vi "PicoScope2000aGetRapidBlock.vi"(0 "error in":errorcluster, 5 "enabled array":i16[](array[numeric]), 7 "handle in":i16, 9 "Buffer and Transfer Settings":T1={"startIndex"=0, "Samples"=1000, "Down Sample Ratio"=2, "Down-Sample Mode"=0} {"Down-Sample Mode" items=["None"=0, "Aggregate"=1, "Decimate"=2, "Average"=4]; "Samples" format="%_6p"}, 11 "Rapid Block Acquisition Settings":T3={"preTriggerSamples"=0, "postTriggerSamples"=1000, "timebase"=2, "Oversample"=1, "Number of Captures"=1}, 12 "Device Info":T2) -> (1 "Channel A Buffer":i16[][](array[numeric]), 2 "Channel B Buffer":i16[][](array[numeric]), 3 "Channel D Buffer":i16[][](array[numeric]), 4 "error out":errorcluster, 6 "handle out":i16, 8 "Port 1":i16[][](array[numeric]), 10 "noOfSamples":u32[](array[numeric]), 13 "Channel C Buffer":i16[][](array[numeric]), 14 "Port 0":i16[][](array[numeric]), 15 "Overflow (binary)":i16[](array[numeric]) format="%06b")   [LabVIEW 2016]
doc: "This VI gets a set of blocks captured using rapid block mode. It outputs two-dimensional arrays for each channel that contain data from all the requested captures."
uses:
  ps2000a.dll
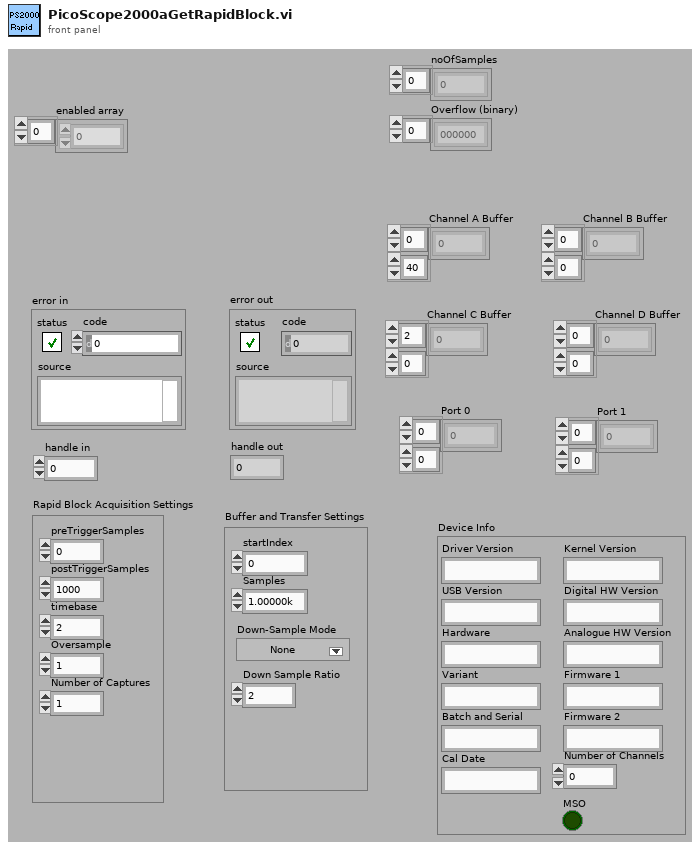
[diagram p1: front panel]
types:
  T1 = cluster{"startIndex":u64, "Samples":u64, "Down Sample Ratio":u64, "Down-Sample Mode":u32}
  T2 = cluster{"Driver Version":string, "USB Version":string, "Hardware":string, "Variant":string, "Batch and Serial":string, "Cal Date":string, "Kernel Version":string, "Digital HW Version":string, "Analogue HW Version":string, "Firmware 1":string, "Firmware 2":string, "MSO":bool, "Number of Channels":i16}
  T3 = cluster{"preTriggerSamples":u32, "postTriggerSamples":u32, "timebase":u32, "Oversample":i16, "Number of Captures":u32}
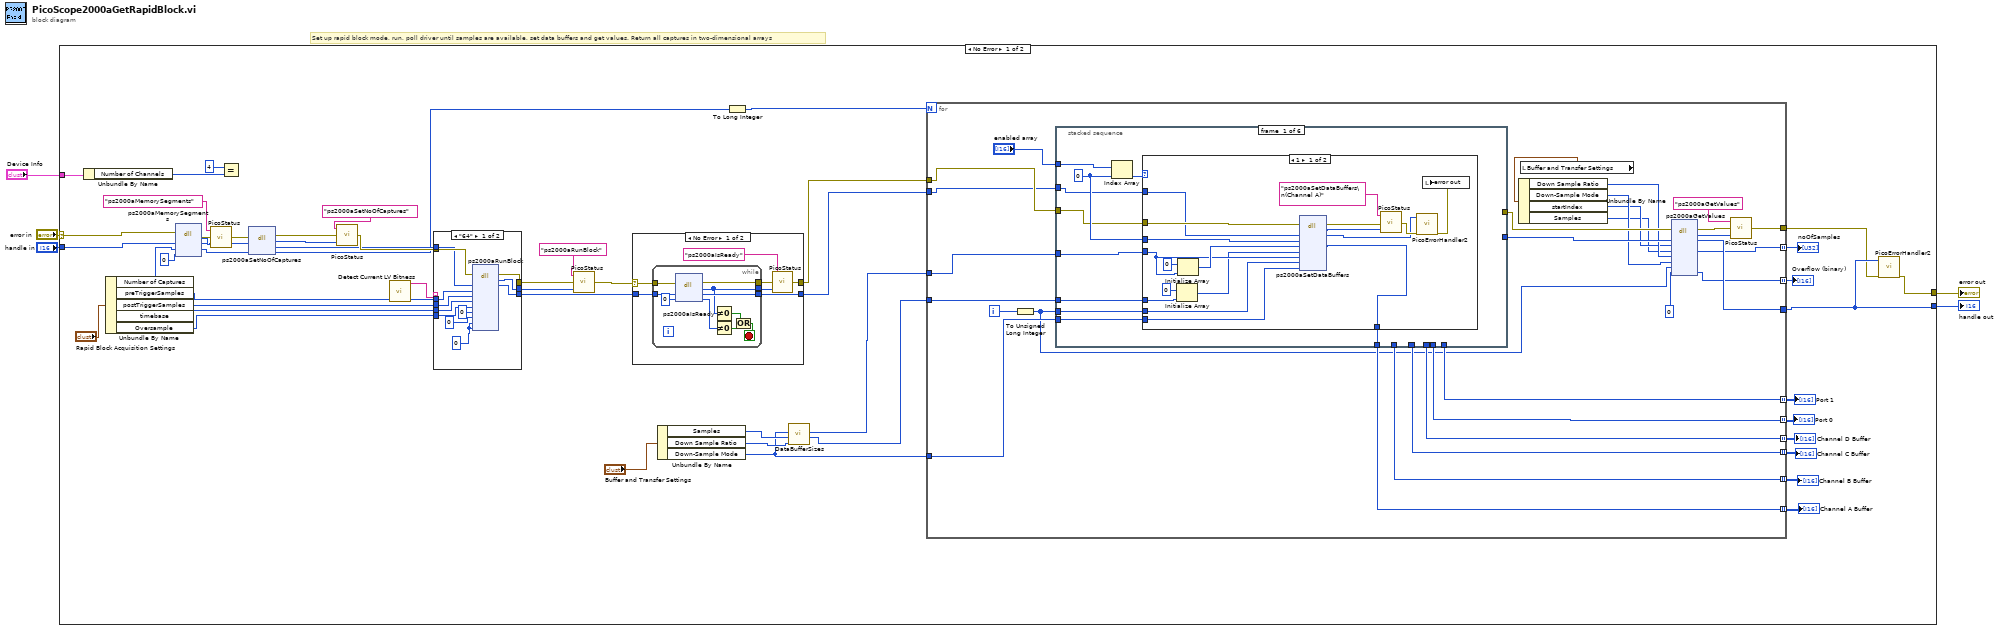
[diagram p0: block diagram]
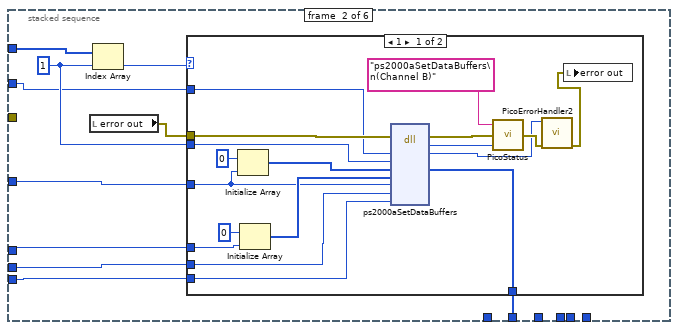
[diagram p3: hidden frame]
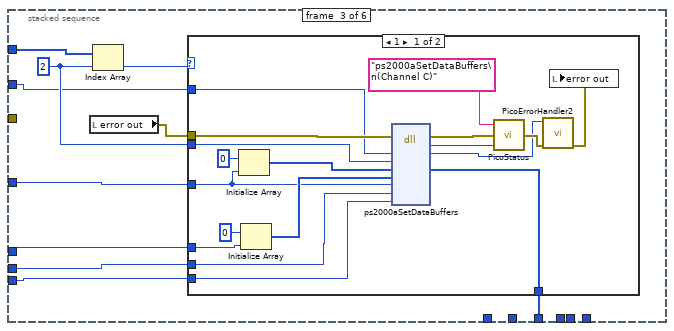
[diagram p5: hidden frame]
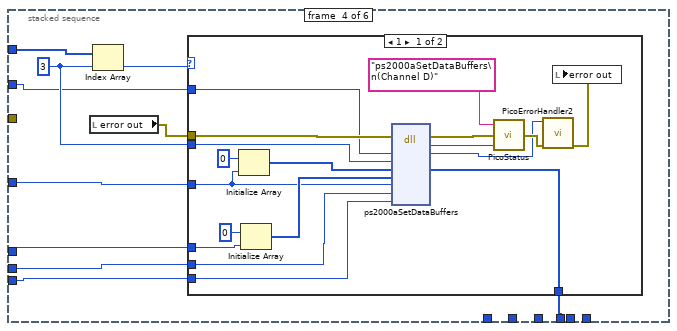
[diagram p7: hidden frame]
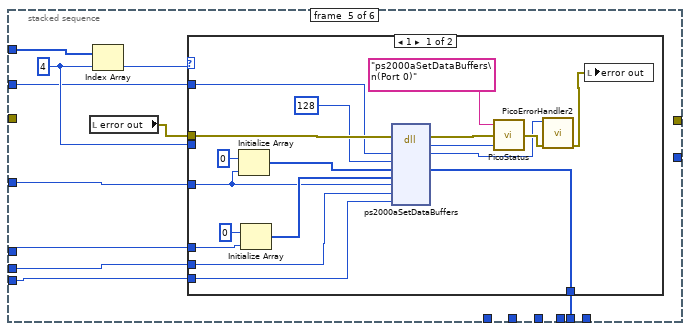
[diagram p9: hidden frame]
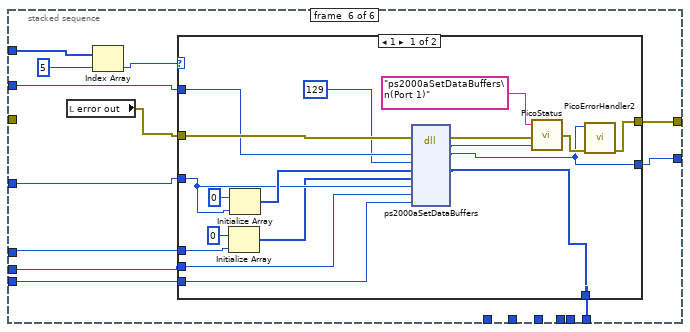
[diagram p11: hidden frame]
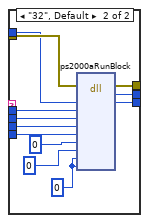
[diagram p13: hidden frame]
diagram:
  # "Set up rapid block mode, run, poll driver until samples are available, set data buffers and get values. Return all captures in two-dimensional arrays"
  n1 = case shown="No Error" "error in" {
    selector: "error in" -> [w45 w301]
    tunnel: [w26 w301] -> w4
    tunnel: "handle in" -> [w44 w300]
    tunnel: [w15 w300] -> w2
    tunnel: "Device Info" -> [w30 _]
    frame No Error {
      n2 = Unbundle By Name(w30) -> ("Number of Channels"=w29:i16)
      n3 = Unbundle By Name("Rapid Block Acquisition Settings") -> ("Number of Captures"=w40:u32, "preTriggerSamples"=w52:u32, "postTriggerSamples"=w51:u32, "timebase"=w53:u32, "Oversample"=w46:i16)
      n4 = dll-call lib="ps2000a.dll" fn="ps2000aMemorySegments" ("ps3000.dll:_ps3000_open_unit@0")(error in=w45, "handle"=w44, "nSegments"=w40, "nMaxSamples"=u32 0) -> (error out=w42:errorcluster, "PICO_STATUS"=w43:i32, "handle"=w37:i16, "nSegments"=w38:u32)  [unwired: 3 in, 1 out]
      n5 = call "PicoStatus.vi"("PICO STATUS"=w43, "error in"=w42, "source"="ps2000aMemorySegments") -> ("error out"=w36:errorcluster)
      n6 = Equal?(x=i16 4, y=w29) -> ()  [unwired: 1 out]
      n7 = dll-call lib="ps2000a.dll" fn="ps2000aSetNoOfCaptures" ("ps3000.dll:_ps3000_open_unit@0")(error in=w36, "handle"=w37, "nCaptures"=w38) -> (error out=w34:errorcluster, "PICO_STATUS"=w35:i32, "handle"=w31:i16, "nCaptures"=w16:u16)  [unwired: 2 in, 1 out]
      n8 = call "PicoStatus.vi"("PICO STATUS"=w35, "error in"=w34, "source"="ps2000aSetNoOfCaptures") -> ("error out"=w32:errorcluster)
      n9 = call "Detect Current LV Bitness.vi"() -> ("bitness"=w27:string)  [unwired: 11 in]
      n10 = case shown="\"64\"" w27 {
        tunnel: [w260 w280] -> w55
        tunnel: w53 -> [w263 w279]
        tunnel: w52 -> [w266 w278]
        tunnel: w51 -> [w265 w277]
        tunnel: [w261 w276] -> w50
        tunnel: [w262 w275] -> w49
        tunnel: w46 -> [w264 w274]
        tunnel: w32 -> [w268 w273]
        tunnel: w31 -> [w267 w272]
        frame "64" {
          w257 = u64 0 ("pParameter")
          n11 = dll-call lib="ps2000a.dll" fn="ps2000aRunBlock" ("ps3000.dll:_ps3000_open_unit@0")(error in=w268, "handle"=w267, "preTriggerSamples"=w266, "postTriggerSamples"=w265, "timebase"=w263, "oversample"=w264, "timeindisposed"=0, "segmentIndex"=u32 0, "lpReady"=w257, "pParameter"=w257) -> (error out=w262:errorcluster, "PICO_STATUS"=w261:i32, "handle"=w260:i16)  [unwired: 10 in, 1 out]
        }
        frame "32", Default {
          w269 = u32 0 ("pParameter")
          n12 = dll-call lib="ps2000a.dll" fn="ps2000aRunBlock" ("ps3000.dll:_ps3000_open_unit@0")(error in=w273, "handle"=w272, "preTriggerSamples"=w278, "postTriggerSamples"=w277, "timebase"=w279, "oversample"=w274, "timeindisposed"=0, "segmentIndex"=u32 0, "lpReady"=w269, "pParameter"=w269) -> (error out=w275:errorcluster, "PICO_STATUS"=w276:i32, "handle"=w280:i16)  [unwired: 10 in, 1 out]
        }
      }
      n13 = call "PicoStatus.vi"("PICO STATUS"=w50, "error in"=w49, "source"="ps2000aRunBlock") -> ("error out"=w48:errorcluster)
      n14 = case shown="No Error" w48 {
        selector: w48 -> [w285 w298]
        tunnel: w55 -> [w287 w299]
        tunnel: [w286 w299] -> w22
        tunnel: [w284 w298] -> w23
        frame No Error {
          n15 = while {
            tunnel: [w297] -> w286
            tunnel: w287 -> [w296]
            tunnel: [w291] -> w282
            tunnel: w285 -> [w290]
            tunnel: [w289] -> w283
            stop <- w295 stop-if-true
            n16 = dll-call lib="ps2000a.dll" fn="ps2000aIsReady" ("ps3000.dll:_ps3000_open_unit@0")(error in=w290, "handle"=w296, "ready"=i16 0) -> (error out=w289:errorcluster, "status"=w291:i32, "handle"=w297:i16, "ready"=w292:i16)  [unwired: 2 in, 1 out]
            n17 = Not Equal To 0?(x=w291) -> (x != 0?=w293:bool)
            n18 = Not Equal To 0?(x=w292) -> (x != 0?=w294:bool)
            n19 = Or(x=w293, y=w294) -> (x .or. y?=w295:bool)
          }
          n20 = call "PicoStatus.vi"("PICO STATUS"=w282, "error in"=w283, "source"="ps2000aIsReady") -> ("error out"=w284:errorcluster)
        }
        frame Error {
        }
      }
      n21 = Unbundle By Name("Buffer and Transfer Settings") -> ("Samples"=w24:u64, "Down Sample Ratio"=w19:u64, "Down-Sample Mode"=w18:u32)
      n22 = To Long Integer(number=w16) -> (32bit integer=w17:i32)
      n23 = call "DataBufferSizes.vi"("Down Sample Ratio"=w19, "Number of Samples"=w24, "Down-Sample Mode"=w18) -> ("min Buffer Size"=w21:i32, "Max Buffer Size"=w20:i32)  [unwired: 7 in]
      n24 = for {
        N: w17 -> [_]
        tunnel: w22 -> [w81]
        tunnel: w23 -> [w82]
        tunnel: w20 -> [w83]
        tunnel: w21 -> [w80]
        tunnel: w18 -> [w79]
        tunnel: [w75] -> w15
        tunnel: [w74] -> w7 mode=indexing
        tunnel: [w73] -> w14 mode=indexing
        tunnel: [w72] -> w13 mode=indexing
        tunnel: [w71] -> w12 mode=indexing
        tunnel: [w70] -> w11 mode=indexing
        tunnel: [w69] -> w10 mode=indexing
        tunnel: [w68] -> w9 mode=indexing
        tunnel: [w64] -> w8
        tunnel: [w58] -> w6 mode=indexing
        i -> [w65]
        n25 = To Unsigned Long Integer(number=w65) -> (unsigned 32bit integer=w62:u32)
        n26 = stacked-sequence {
          tunnel: "enabled array" -> [w93 w121 w149 w177 w205 w235]
          tunnel: w82 -> [w91 _ _ _ _ _]
          tunnel: w81 -> [w90 w119 w147 w175 w197 w232]
          tunnel: w83 -> [w87 w118 w146 w174 w204 w229]
          tunnel: [w89 _ _ _ _ _] -> w73
          tunnel: w62 -> [w88 w117 w145 w173 w203 w231]
          tunnel: [_ w116 _ _ _ _] -> w72
          tunnel: [_ _ w141 _ _ _] -> w71
          tunnel: [_ _ _ w169 _ _] -> w70
          tunnel: [_ _ _ _ w199 _] -> w69
          tunnel: [_ _ _ _ _ w228] -> w68
          tunnel: w80 -> [w86 w114 w143 w171 w201 w230]
          tunnel: w79 -> [w85 w113 w142 w170 w200 w227]
          tunnel: [_ _ _ _ _ w226] -> w67
          tunnel: [_ _ _ _ _ w225] -> w66
          frame #0 {
            w94 = 0 ("dimension size")
            n27 = Index Array(array=w93, index=w94) -> (element=w92:i16)
            n28 = case shown="1" w92 {
              tunnel: w94 -> [w106 _]
              tunnel: w91 -> [w108 _]
              tunnel: w90 -> [w107 _]
              tunnel: w87 -> [w104 _]
              tunnel: [w99 _] -> w89
              tunnel: w88 -> [w103 _]
              tunnel: w86 -> [w98 _]
              tunnel: w85 -> [w95 _]
              frame 1 {
                n29 = Initialize Array(i16 0 ("element"), w98) -> (w97:i16[])
                n30 = Initialize Array(i16 0 ("element"), w104) -> (w105:i16[])
                n31 = dll-call lib="ps2000a.dll" fn="ps2000aSetDataBuffers" ("ps3000.dll:_ps3000_open_unit@0")(error in=w108, "handle"=w107, "channel"=w106, "bufferMax"=w105, "bufferMin"=w97, "bufferLth"=w104, "segmentIndex"=w103, "downSampleRatioMode"=w95) -> (error out=w102:errorcluster, "PICO_STATUS"=w101:i32, "handle"=w100:i16, "bufferMax"=w99:i16[])  [unwired: 7 in, 1 out]
                n32 = call "PicoStatus.vi"("PICO STATUS"=w101, "error in"=w102, "source"="ps2000aSetDataBuffers\n(Channel A)") -> ("error out"=w111:errorcluster)
                n33 = call "PicoErrorHandler2.vi"("error in (no error)"=w111, "handle In"=w100) -> ("error out"=w110:errorcluster)  [unwired: 9 in]
                n34 = local write "error out"(w110) -> ()
              }
              frame 0, Default {
              }
            }
          }
          frame #1 {
            w122 = 1 ("dimension size")
            n35 = local read "error out"() -> (w115:errorcluster)
            n36 = Index Array(array=w121, index=w122) -> (element=w120:i16)
            n37 = case shown="1" w120 {
              tunnel: w122 -> [w126 _]
              tunnel: w115 -> [w131 _]
              tunnel: w119 -> [w123 _]
              tunnel: w118 -> [w129 _]
              tunnel: [w125 _] -> w116
              tunnel: w117 -> [w130 _]
              tunnel: w114 -> [w128 _]
              tunnel: w113 -> [w124 _]
              frame 1 {
                n38 = Initialize Array(i16 0 ("element"), w129) -> (w138:i16[])
                n39 = Initialize Array(i16 0 ("element"), w128) -> (w137:i16[])
                n40 = dll-call lib="ps2000a.dll" fn="ps2000aSetDataBuffers" ("ps3000.dll:_ps3000_open_unit@0")(error in=w131, "handle"=w123, "channel"=w126, "bufferMax"=w138, "bufferMin"=w137, "bufferLth"=w129, "segmentIndex"=w130, "downSampleRatioMode"=w124) -> (error out=w135:errorcluster, "PICO_STATUS"=w133:i32, "handle"=w132:i16, "bufferMax"=w125:i16[])  [unwired: 7 in, 1 out]
                n41 = call "PicoStatus.vi"("PICO STATUS"=w133, "error in"=w135, "source"="ps2000aSetDataBuffers\n(Channel B)") -> ("error out"=w139:errorcluster)
                n42 = call "PicoErrorHandler2.vi"("error in (no error)"=w139, "handle In"=w132) -> ("error out"=w140:errorcluster)  [unwired: 9 in]
                n43 = local write "error out"(w140) -> ()
              }
              frame 0, Default {
              }
            }
          }
          frame #2 {
            w150 = 2 ("dimension size")
            n44 = local read "error out"() -> (w144:errorcluster)
            n45 = Index Array(array=w149, index=w150) -> (element=w148:i16)
            n46 = case shown="1" w148 {
              tunnel: w150 -> [w154 _]
              tunnel: w144 -> [w159 _]
              tunnel: w147 -> [w151 _]
              tunnel: w146 -> [w157 _]
              tunnel: [w153 _] -> w141
              tunnel: w145 -> [w158 _]
              tunnel: w143 -> [w156 _]
              tunnel: w142 -> [w152 _]
              frame 1 {
                n47 = Initialize Array(i16 0 ("element"), w157) -> (w166:i16[])
                n48 = Initialize Array(i16 0 ("element"), w156) -> (w165:i16[])
                n49 = dll-call lib="ps2000a.dll" fn="ps2000aSetDataBuffers" ("ps3000.dll:_ps3000_open_unit@0")(error in=w159, "handle"=w151, "channel"=w154, "bufferMax"=w166, "bufferMin"=w165, "bufferLth"=w157, "segmentIndex"=w158, "downSampleRatioMode"=w152) -> (error out=w163:errorcluster, "PICO_STATUS"=w161:i32, "handle"=w160:i16, "bufferMax"=w153:i16[])  [unwired: 7 in, 1 out]
                n50 = call "PicoStatus.vi"("PICO STATUS"=w161, "error in"=w163, "source"="ps2000aSetDataBuffers\n(Channel C)") -> ("error out"=w167:errorcluster)
                n51 = call "PicoErrorHandler2.vi"("error in (no error)"=w167, "handle In"=w160) -> ("error out"=w168:errorcluster)  [unwired: 9 in]
                n52 = local write "error out"(w168) -> ()
              }
              frame 0, Default {
              }
            }
          }
          frame #3 {
            w178 = 3 ("dimension size")
            n53 = local read "error out"() -> (w172:errorcluster)
            n54 = Index Array(array=w177, index=w178) -> (element=w176:i16)
            n55 = case shown="1" w176 {
              tunnel: w178 -> [w182 _]
              tunnel: w172 -> [w187 _]
              tunnel: w175 -> [w179 _]
              tunnel: w174 -> [w185 _]
              tunnel: [w181 _] -> w169
              tunnel: w173 -> [w186 _]
              tunnel: w171 -> [w184 _]
              tunnel: w170 -> [w180 _]
              frame 1 {
                n56 = Initialize Array(i16 0 ("element"), w185) -> (w194:i16[])
                n57 = Initialize Array(i16 0 ("element"), w184) -> (w193:i16[])
                n58 = dll-call lib="ps2000a.dll" fn="ps2000aSetDataBuffers" ("ps3000.dll:_ps3000_open_unit@0")(error in=w187, "handle"=w179, "channel"=w182, "bufferMax"=w194, "bufferMin"=w193, "bufferLth"=w185, "segmentIndex"=w186, "downSampleRatioMode"=w180) -> (error out=w191:errorcluster, "PICO_STATUS"=w189:i32, "handle"=w188:i16, "bufferMax"=w181:i16[])  [unwired: 7 in, 1 out]
                n59 = call "PicoStatus.vi"("PICO STATUS"=w189, "error in"=w191, "source"="ps2000aSetDataBuffers\n(Channel D)") -> ("error out"=w195:errorcluster)
                n60 = call "PicoErrorHandler2.vi"("error in (no error)"=w195, "handle In"=w188) -> ("error out"=w196:errorcluster)  [unwired: 9 in]
                n61 = local write "error out"(w196) -> ()
              }
              frame 0, Default {
              }
            }
          }
          frame #4 {
            w206 = 4 ("dimension size")
            n62 = local read "error out"() -> (w202:errorcluster)
            n63 = Index Array(array=w205, index=w206) -> (element=w198:i16)
            n64 = case shown="1" w198 {
              tunnel: w206 -> [_ _]
              tunnel: w202 -> [w215 _]
              tunnel: w204 -> [w213 _]
              tunnel: [w210 _] -> w199
              tunnel: w203 -> [w214 _]
              tunnel: w201 -> [w212 _]
              tunnel: w200 -> [w209 _]
              tunnel: w197 -> [w207 _]
              frame 1 {
                n65 = Initialize Array(i16 0 ("element"), w213) -> (w222:i16[])
                n66 = Initialize Array(i16 0 ("element"), w212) -> (w221:i16[])
                n67 = dll-call lib="ps2000a.dll" fn="ps2000aSetDataBuffers" ("ps3000.dll:_ps3000_open_unit@0")(error in=w215, "handle"=w207, "channel"=128, "bufferMax"=w222, "bufferMin"=w221, "bufferLth"=w213, "segmentIndex"=w214, "downSampleRatioMode"=w209) -> (error out=w219:errorcluster, "PICO_STATUS"=w217:i32, "handle"=w216:i16, "bufferMax"=w210:i16[])  [unwired: 7 in, 1 out]
                n68 = call "PicoStatus.vi"("PICO STATUS"=w217, "error in"=w219, "source"="ps2000aSetDataBuffers\n(Port 0)") -> ("error out"=w223:errorcluster)
                n69 = call "PicoErrorHandler2.vi"("error in (no error)"=w223, "handle In"=w216) -> ("error out"=w224:errorcluster)  [unwired: 9 in]
                n70 = local write "error out"(w224) -> ()
              }
              frame 0, Default {
              }
            }
          }
          frame #5 {
            n71 = local read "error out"() -> (w234:errorcluster)
            n72 = Index Array(array=w235, index=5 ("dimension size")) -> (element=w233:i16)
            n73 = case shown="1" w233 {
              tunnel: w234 -> [w251 w256]
              tunnel: w232 -> [w250 w255]
              tunnel: w229 -> [w248 _]
              tunnel: [w244 _] -> w228
              tunnel: w231 -> [w247 _]
              tunnel: w230 -> [w243 _]
              tunnel: [w240 w256] -> w226
              tunnel: [w239 w255] -> w225
              tunnel: w227 -> [w237 _]
              frame 1 {
                n74 = Initialize Array(i16 0 ("element"), w243) -> (w242:i16[])
                n75 = Initialize Array(i16 0 ("element"), w248) -> (w249:i16[])
                n76 = dll-call lib="ps2000a.dll" fn="ps2000aSetDataBuffers" ("ps3000.dll:_ps3000_open_unit@0")(error in=w251, "handle"=w250, "channel"=129, "bufferMax"=w249, "bufferMin"=w242, "bufferLth"=w248, "segmentIndex"=w247, "downSampleRatioMode"=w237) -> (error out=w246:errorcluster, "PICO_STATUS"=w245:u32, "handle"=w239:i16, "bufferMax"=w244:i16[])  [unwired: 7 in, 1 out]
                n77 = call "PicoStatus.vi"("PICO STATUS"=w245, "error in"=w246, "source"="ps2000aSetDataBuffers\n(Port 1)") -> ("error out"=w253:errorcluster)
                n78 = call "PicoErrorHandler2.vi"("error in (no error)"=w253, "handle In"=w239) -> ("error out"=w240:errorcluster)  [unwired: 9 in]
              }
              frame 0, Default {
              }
            }
          }
        }
        n79 = local read "Buffer and Transfer Settings"() -> (w61:T1)
        n80 = Unbundle By Name(w61) -> ("Down Sample Ratio"=w60:u64, "Down-Sample Mode"=w59:u32, "startIndex"=w57:u64, "Samples"=w56:u64)
        n81 = dll-call lib="ps2000a.dll" fn="ps2000aGetValues" ("ps3000.dll:_ps3000_open_unit@0")(error in=w67, "handle"=w66, "startIndex"=w57, "noOfSamples"=w56, "downSampleRatio"=w60, "downSampleRatioMode"=w59, "SegmentIndex"=w62, "overflow"=i16 0) -> (error out=w77:errorcluster, "PICO_STATUS"=w78:u32, "handle"=w75:i16, "noOfSamples"=w74:u32, "overflow"=w58:i16)  [unwired: 6 in, 1 out]
        n82 = call "PicoStatus.vi"("PICO STATUS"=w78, "error in"=w77, "source"="ps2000aGetValues") -> ("error out"=w64:errorcluster)
      }
      "Channel D Buffer" <- w11
      "Channel C Buffer" <- w12
      "Channel B Buffer" <- w13
      "Channel A Buffer" <- w14
      "Port 0" <- w10
      "Port 1" <- w9
      "noOfSamples" <- w7
      "Overflow (binary)" <- w6
      n83 = call "PicoErrorHandler2.vi"("error in (no error)"=w8, "handle In"=w15) -> ("error out"=w26:errorcluster)  [unwired: 9 in]
    }
    frame Error {
    }
  }
  "error out" <- w4
  "handle out" <- w2
